vi "Jpeg file pattern.vi"(3 "error in":errorcluster) -> (6 "path to JPG file":path, 9 "error out":errorcluster)   [LabVIEW 2013]
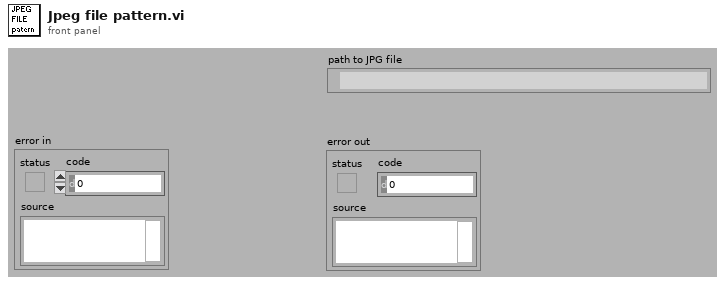
[diagram p1: front panel]
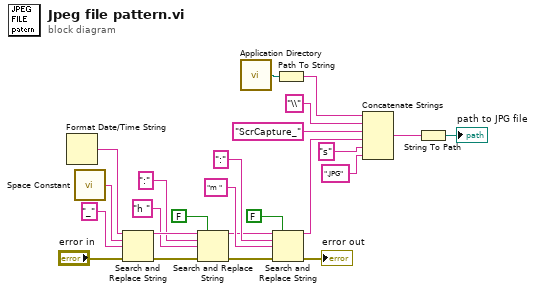
[diagram p0: block diagram]
diagram:
  n1 = Format Date/Time String() -> (date/time string=w24:string)  [unwired: 3 out]
  n2 = call <vilib>:"Space Constant.vi"() -> ("String"=w23:string)
  n3 = Search and Replace String(input string=w24, search string=w23, replace string="_" ("replace string (\"\")"), error in="error in") -> (result string=w22:string, error out=w13:errorcluster)  [unwired: 6 out]
  n4 = Search and Replace String(replace all?=FALSE ("replace all? (F)"), input string=w22, search string=":", replace string="h " ("replace string (\"\")"), error in=w13) -> (result string=w15:string, error out=w12:errorcluster)  [unwired: 5 out]
  n5 = call <vilib>:"Application Directory.vi"() -> ("Application Directory"=w3:path)
  n6 = Search and Replace String(replace all?=FALSE ("replace all? (F)"), input string=w15, search string=":", replace string="m " ("replace string (\"\")"), error in=w12) -> (result string=w7:string, error out=→"error out":errorcluster)  [unwired: 5 out]
  n7 = Path To String(path=w3) -> (string=w5:string)
  n8 = Concatenate Strings(w5, "\\" ("string"), "ScrCapture_" ("string"), w7, "s" ("string"), ".JPG" ("default name")) -> (w11:string)
  n9 = String To Path(string=w11) -> (path=→"path to JPG file":path)
